vi "Periodic Tasks.vi"(8 "error in":errorcluster) -> ()   [LabVIEW 2016]
doc: "This VI runs in parallel to other tasks. It can contain as many user-defined periodic loops as you need. These can carry out PID or other sorts of timed response."
uses:
  Refname/Motors.ctl
  Refname/Sensors.ctl
  Refname/Queues.ctl
  <vilib>/Rock Robotics/WPI/DriverStation/WPI_DriverStationRobotMode2.ctl
  Refname/Refname to String (Motors).vi
  Robot Global Data.vi
  Refname/Refname to String (Sensors).vi
panel:
  in  "Low Sensitivity z":dbl=1.9 format="%#_13g"
  in  "Default Sensitivity z":dbl=1.6 format="%#_13g"
  in  "Low Sensitivity x & y":dbl=1.7 format="%#_13g"
  in  "Default Sensitivity x & y":dbl=1.4 format="%#_13g"
  out "error out":errorcluster
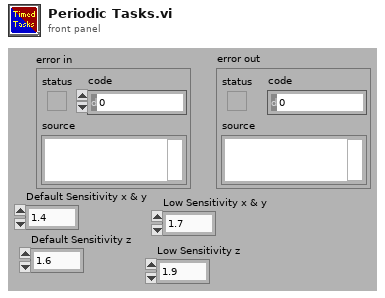
[diagram p1: front panel]
types:
  T1 = typedef "Queues.ctl" = enum16{"Log Queue"}
  T2 = typedef "Sensors.ctl" = enum16{"DIP 1", "DIP 2", "DIP 3", "DIP 4", "IMU", "HuskieBoard"}
  T3 = typedef "Motors.ctl" = enum16{"Wheel 1", "Swerve 1", "Wheel 2", "Swerve 2", "Wheel 3", "Swerve 3", "Wheel 4", "Swerve 4", "Climber"}
  T4 = typedef "WPI_MotorControlDeviceRef.ctl" = cluster{"DeviceStatus":errorcluster, "Type":T5, "PWM":cluster{"PWM Channel":T6, "DeadBand":T7}, "CAN":cluster{"Device Number":u8, "SetOutput VI Ref":variant, "GetOutput VI Ref":variant, "Enable VI Ref":variant, "Disable VI Ref":variant, "Data":variant}, "Invert":bool}
  T5 = typedef "WPI_MotorControlType.ctl" = enum16{"PWM", "CAN"}
  T6 = typedef "FPGA_DIOPWMChannel.ctl" = enum8{"PWM 0", "PWM 1", "PWM 2", "PWM 3", "PWM 4", "PWM 5", "PWM 6", "PWM 7", "PWM 8", "PWM 9", "PWM MXP 0", "PWM MXP 1", "PWM MXP 2", "PWM MXP 3", "PWM MXP 4", "PWM MXP 5", "PWM MXP 6", "PWM MXP 7", "PWM MXP 8", "PWM MXP 9", "Invalid"}
  T7 = typedef "WPI_PWMDeadband.ctl" = cluster{"Name":string, "maxPositivePwm":i32, "minPositivePwm":i32, "centerPwm":i32, "maxNegativePwm":i32, "minNegativePwm":i32, "angularRange":u16}
  T8 = typedef "WPI_SerialPortRef.ctl" = cluster{"DevStatus":errorcluster, "Serial Port Name":refnum<visa-resource-name>}
  T9 = enum8{"Don't Change", "Backlight On", "Backlight Off"}
  T10 = typedef "WPI_CANTalonSRX_GlobalStatus.ctl" = cluster{"Applied Throttle":dbl, "Module Enabled":bool, "CAN Error":errorcluster, "Closed Loop Error":dbl, "Forward Limit Switch Closed":bool, "Reverse Limit Switch Closed":bool, "Sensor Position":dbl, "Sensor Velocity":dbl, "Current":dbl, "Sticky Fault - Over Temp":bool, "Sticky Fault - Under Voltage":bool, "Sticky Fault - Forward Limit":bool, "Sticky Fault - Reverse Limit":bool, "Sticky Fault - Forward Soft Limit":bool, "Sticky Fault - Reverse Soft Limit":bool, "Brake is Enabled":bool, "Encoder Position":dbl, "Encoder Velocity":dbl, "Encoder Index Count":dbl, "Encoder A Pin State":bool, "Encoder B Pin State":bool, "Encoder Index Pin State":bool, "Analog In":dbl, "Analog In Velocity":dbl, "Temperature (C)":dbl, "Battery Voltage":dbl, "Control 5 Is Supported":bool, "Current Profile Slot Select":dbl, "Pos Div 8":bool, "Vel Div 4":bool, "Pulse Width Position":i32, "Pulse Width Velocity":i32, "Pulse Width Rise To Rise (us)":i32, "Pulse Width Rise To Fall (us)":i32, "Mot Prof Active Is Under Run":bool, "Mot Prof Active Has Under Run":bool, "Mot Prof Active Is Last":bool, "Mot Prof Active Velocity Only":bool, "Mot Prof Active Is Valid":bool, "Mot Prof Buffer Is Full":bool, "Mot Prof Active Profile Slot Select":i32, "Mot Prof NextID":i32, "Mot Prof Count":i32, "Mot Prof Active Velocity":dbl, "Mot Prof Active Position":dbl, "Mot Prof Output Enable":i32}
  T11 = cluster{"X":dbl, "Y":dbl, "Z":dbl, "B (Straight Drive)":bool, "T1 (Climber Up)":bool, "T2 (Climber Down)":bool, "Pinky Trigger (Low Sensitivity Drive)":bool, "Trigger Full Press (Reverse Drive)":bool, "LED Green":bool}
  T12 = typedef "WPI_DriverStationRobotMode2.ctl" = enum16{"Autonomous Disabled", "Autonomous Enabled", "Teleop Disabled", "Teleop Enabled", "Disconnected", "Finish", "Test Disabled", "Test Enabled", "Emergency Stopped"}
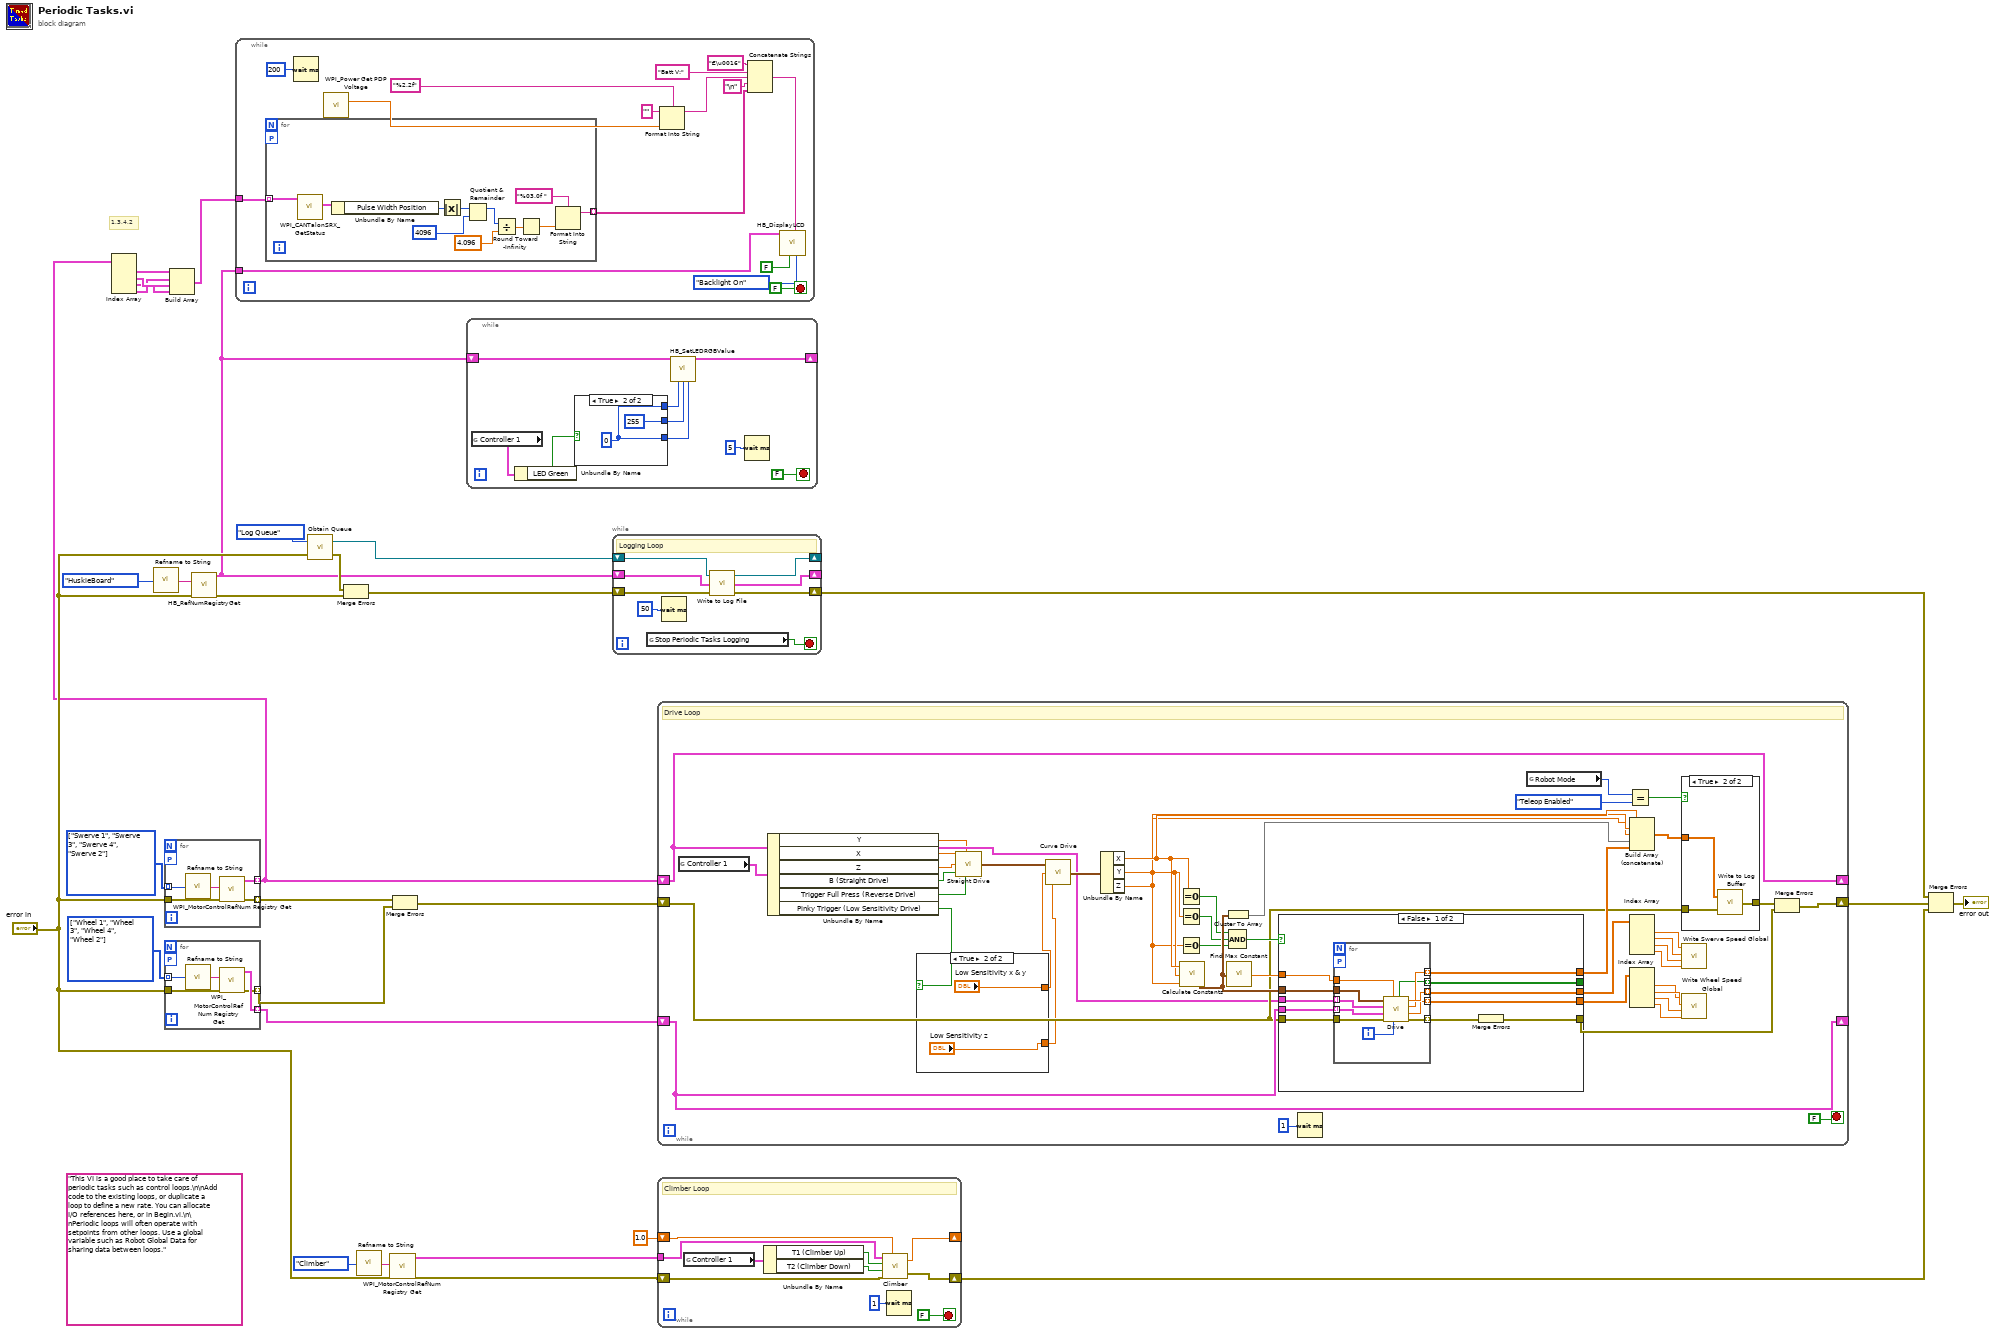
[diagram p0: block diagram]
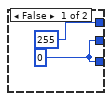
[diagram p2: hidden frame]
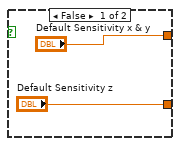
[diagram p3: hidden frame]
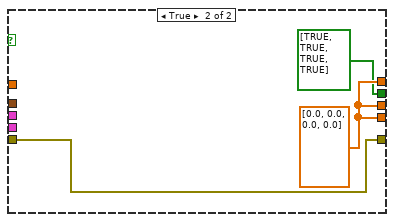
[diagram p4: hidden frame]
diagram:
  w28 = T3[] [enum."Wheel 1", enum."Wheel 3", enum."Wheel 4", enum."Wheel 2"] items=["Wheel 1", "Swerve 1", "Wheel 2", "Swerve 2", "Wheel 3", "Swerve 3", "Wheel 4", "Swerve 4", "Climber"]
  w29 = T3[] [enum."Swerve 1", enum."Swerve 3", enum."Swerve 4", enum."Swerve 2"] items=["Wheel 1", "Swerve 1", "Wheel 2", "Swerve 2", "Wheel 3", "Swerve 3", "Wheel 4", "Swerve 4", "Climber"]
  (unwired) "This VI is a good place to take care of periodic tasks such as control loops.\n\nAdd code to the existing loops, or duplicate a loop to define a new rate. You can allocate I/O references here, or in Begin.vi.\n\nPeriodic loops will often operate with setpoints from other loops. Use a global variable such as Robot Global Data for sharing data between loops."
  # "1,3,4,2"
  n1 = call-poly "Refname to String.vi"("Enum"=Sensors."HuskieBoard") -> ("String"=w17:string)
  n2 = for {
    tunnel: [w35] -> w6 mode=indexing
    tunnel: w29 -> [w33] mode=indexing
    workers-P: _ -> [_]
    tunnel: "error in" -> [w32]
    tunnel: [w31] -> w26 mode=indexing
    n3 = call-poly "Refname to String.vi"("Enum"=w33) -> ("String"=w34:string)
    n4 = call <vilib>:"WPI_MotorControlRefNum Registry Get.vi"("error in (no error)"=w32, "refnum name"=w34) -> ("error out"=w31:errorcluster, "MotorControlDevRef"=w35:T4)  [unwired: 8 in]
  }
  n5 = Index Array(array=w6) -> (element #1=w5:T4, element #2=w4:T4, element #3=w3:T4, element #4=w2:T4)  [unwired: 4 in]
  n6 = for {
    tunnel: [w40] -> w30 mode=indexing
    tunnel: w28 -> [w38] mode=indexing
    workers-P: _ -> [_]
    tunnel: "error in" -> [w37]
    tunnel: [w36] -> w25 mode=indexing
    n7 = call-poly "Refname to String.vi"("Enum"=w38) -> ("String"=w39:string)
    n8 = call <vilib>:"WPI_MotorControlRefNum Registry Get.vi"("error in (no error)"=w37, "refnum name"=w39) -> ("error out"=w36:errorcluster, "MotorControlDevRef"=w40:T4)  [unwired: 8 in]
  }
  n9 = Build Array(w5, w2, w4, w3) -> (w1:T4[])
  n10 = call <vilib>:"HB_RefNumRegistryGet.vi"("refnum name"=w17, "error in (no error)"="error in") -> ("HBDevRef"=w7:T8, "error out"=w11:errorcluster)  [unwired: 12 in]
  n11 = while {
    tunnel: w7 -> [w53]
    tunnel: w1 -> [w42]
    stop <- FALSE stop-if-true
    n12 = for {
      tunnel: w42 -> [w66] mode=indexing
      workers-P: _ -> [_]
      tunnel: [w57] -> w41 mode=indexing
      n13 = call <vilib>:"WPI_CANTalonSRX_GetStatus.vi"("CAN Talon SRX Ref"=w66) -> ("Talon SRX Status"=w65:T10)  [unwired: 8 in, 2 out]
      n14 = Unbundle By Name(w65) -> ("Pulse Width Position"=w64:i32)
      n15 = Absolute Value(x=w64) -> (abs(x)=w63:i32)
      n16 = Quotient & Remainder(x=w63, y=4096) -> (x-y*floor(x/y)=w56:i32)  [unwired: 1 out]
      n17 = Divide(x=w56, y=4.096) -> (x/y=w60:dbl)
      n18 = Round Toward -Infinity(1:w60) -> (0:w58:dbl)
      n19 = Format Into String(format string="%03.0f ", w58) -> (resulting string=w57:string)  [unwired: 2 in, 1 out]
    }
    n20 = Wait (ms)(milliseconds to wait=u32 200) -> ()  [unwired: 1 out]
    n21 = call <vilib>:"WPI_Power Get PDP Voltage.vi"() -> ("voltage (V)"=w49:dbl)  [unwired: 14 in, 1 out]
    n22 = Format Into String(format string="%2.2f", initial string="", w49) -> (resulting string=w47:string)  [unwired: 1 in, 1 out]
    n23 = Concatenate Strings("€\u0016" ("string"), "Batt V:" ("string"), w47, "\n" ("string"), w41) -> (w52:string)
    n24 = call <vilib>:"HB_DisplayLCD.vi"("LCD Backlight"=T9."Backlight On", "Clear LCD Display"=FALSE, "Display String"=w52, "HBDeviceRef"=w53) -> ()  [unwired: 6 in, 2 out]
  }
  n25 = call "Obtain Queue.vi"("error in"="error in", "Queue"=Queues."Log Queue") -> ("error out"=w12:errorcluster, "Queue Ref"=w14:refnum<queue>)
  n26 = Merge Errors(w12, w11) -> (w13:errorcluster)
  n27 = call-poly "Refname to String.vi"("Enum"=Motors."Climber") -> ("String"=w24:string)
  n28 = call <vilib>:"WPI_MotorControlRefNum Registry Get.vi"("error in (no error)"="error in", "refnum name"=w24) -> ("error out"=w21:errorcluster, "MotorControlDevRef"=w22:T4)  [unwired: 8 in]
  n29 = Merge Errors(w26, w25) -> (w19:errorcluster)
  n30 = while {
    shift-right: [w74] -> _
    shift-left: w7 -> [w75]
    stop <- FALSE stop-if-true
    n31 = global read "Robot Global Data.vi" "Controller 1"() -> (w69:T11)
    n32 = Unbundle By Name(w69) -> ("LED Green"=w68:bool)
    n33 = case shown="True" w68 {
      tunnel: [255 w78] -> w73
      tunnel: [w76 255] -> w72
      tunnel: [w76 w78] -> w71
      frame False {
        w76 = 0
      }
      frame True {
        w78 = 0
      }
    }
    n34 = call <vilib>:"HB_SetLEDRGBValue.vi"("HBDevRef"=w75, "Red"=w73, "Green"=w72, "Blue"=w71) -> ("HBDevRef"=w74:T8)  [unwired: 10 in, 1 out]
    n35 = Wait (ms)(milliseconds to wait=u32 5) -> ()  [unwired: 1 out]
  }
  n36 = while {
    shift-right: [w85] -> _
    shift-left: w14 -> [w86]
    shift-right: [w83] -> _
    shift-left: w7 -> [w84]
    shift-right: [w81] -> w10
    shift-left: w13 -> [w82]
    stop <- w87 stop-if-true
    # "Logging Loop"
    n37 = global read "Robot Global Data.vi" "Stop Periodic Tasks Logging"() -> (w87:bool)
    n38 = Wait (ms)(milliseconds to wait=u32 50) -> ()  [unwired: 1 out]
    n39 = call "Write to Log File.vi"("error in"=w82, "HBDevRef"=w84, "Log Queue"=w86) -> ("error out"=w81:errorcluster, "HBDevRef"=w83:T8, "Log Queue"=w85:refnum<queue>)
  }
  n40 = while {
    shift-right: [w97] -> _
    shift-left: w6 -> [w97]
    shift-right: [w129] -> _
    shift-left: w30 -> [w129]
    shift-right: [w112] -> w9
    shift-left: w19 -> [w98]
    stop <- FALSE stop-if-true
    # "Drive Loop"
    n41 = global read "Robot Global Data.vi" "Controller 1"() -> (w93:T11)
    n42 = Unbundle By Name(w93) -> ("Y"=w89:dbl, "X"=w88:dbl, "Z"=w90:dbl, "B (Straight Drive)"=w91:bool, "Trigger Full Press (Reverse Drive)"=w92:bool, "Pinky Trigger (Low Sensitivity Drive)"=w96:bool)
    n43 = case shown="True" w96 {
      tunnel: ["Default Sensitivity x & y" "Low Sensitivity x & y"] -> w95
      tunnel: ["Default Sensitivity z" "Low Sensitivity z"] -> w94
      frame False {
      }
      frame True {
      }
    }
    n44 = call "Straight Drive.vi"("X"=w88, "Y"=w89, "Z"=w90, "Straight?"=w91, "Reverse?"=w92) -> ("Axes Magnitudes"=w99:cluster{"X":dbl, "Y":dbl, "Z":dbl})
    n45 = call "Curve Drive.vi"("z exponent"=w94, "x & y exponent"=w95, "Axes Magnitudes"=w99) -> ("Axes Magnitudes"=w100:cluster{"X":dbl, "Y":dbl, "Z":dbl})
    n46 = Unbundle By Name(w100) -> ("X"=w103:dbl, "Y"=w102:dbl, "Z"=w101:dbl)
    n47 = Equal To 0?(x=w103) -> (x = 0?=w120:bool)
    n48 = Equal To 0?(x=w102) -> (x = 0?=w119:bool)
    n49 = Equal To 0?(x=w101) -> (x = 0?=w118:bool)
    n50 = call "Calculate Constants.vi"("Z"=w101, "Y"=w102, "X"=w103) -> ("constants cluster"=w122:cluster{"a":dbl, "b":dbl, "c":dbl, "d":dbl})
    n51 = Cluster To Array(cluster=w122) -> (array=w108:dbl[])
    n52 = call "Find Max Constant.vi"("constants"=w122) -> ("Max or 1"=w121:dbl)
    n53 = Compound Arithmetic op=AND(w120, w119, w118) -> (w117:bool)
    n54 = case shown="False" w117 {
      tunnel: w129 -> [w146 _]
      tunnel: [w145 w160] -> w126
      tunnel: [w144 w160] -> w125
      tunnel: w98 -> [w143 w159]
      tunnel: w97 -> [w142 _]
      tunnel: w122 -> [w141 _]
      tunnel: w121 -> [w140 _]
      tunnel: [w139 w160] -> w109
      tunnel: [w138 w159] -> w104
      tunnel: [w136 bool[] [TRUE, TRUE, TRUE, TRUE]] -> _
      frame False {
        n55 = for {
          tunnel: w142 -> [w148] mode=indexing
          tunnel: w146 -> [w157] mode=indexing
          tunnel: [w156] -> w145 mode=indexing
          tunnel: [w155] -> w144 mode=indexing
          tunnel: w143 -> [w154]
          tunnel: [w150] -> w137 mode=indexing
          tunnel: w141 -> [w153]
          tunnel: w140 -> [w152]
          tunnel: [w149] -> w139 mode=indexing
          workers-P: _ -> [_]
          tunnel: [w147] -> w136 mode=indexing
          i -> [w151]
          n56 = call "Drive.vi"("Index"=w151, "Max Speed or 1"=w152, "error in"=w154, "Wheel DevRef"=w157, "Swerve DevRef"=w148, "constants"=w153) -> ("error out"=w150:errorcluster, "Wheel Speed"=w155:dbl, "Setpoint"=w149:dbl, "Swerve Speed"=w156:dbl, "Reverse?"=w147:bool)  [unwired: 1 in]
        }
        n57 = Merge Errors(w137) -> (w138:errorcluster)
      }
      frame True {
        w160 = dbl[] [0.0, 0.0, 0.0, 0.0]
      }
    }
    n58 = Wait (ms)(milliseconds to wait=u32 1) -> ()  [unwired: 1 out]
    n59 = global read "Robot Global Data.vi" "Robot Mode"() -> (w105:T12)
    n60 = Equal?(x=w105, y=WPI_DriverStationRobotMode2."Teleop Enabled" ("Robot Mode")) -> (x = y?=w107:bool)
    n61 = Build Array (concatenate)(w103, w102, w101, w108, w109) -> (w110:dbl[])
    n62 = Index Array(array=w126) -> (element #1=w116:dbl, element #2=w115:dbl, element #3=w114:dbl, element #4=w113:dbl)  [unwired: 4 in]
    n63 = Index Array(array=w125) -> (element #1=w127:dbl, element #2=w128:dbl, element #3=w124:dbl, element #4=w123:dbl)  [unwired: 4 in]
    n64 = case shown="True" w107 {
      tunnel: w110 -> [_ w162]
      tunnel: [w161 w164] -> w111
      tunnel: w98 -> [w161 w163]
      frame False {
      }
      frame True {
        n65 = call "Write to Log Buffer.vi"("error in"=w163, "array of values"=w162) -> ("error out"=w164:errorcluster)
      }
    }
    n66 = call "Write Swerve Speed Global.vi"("Swerve 4"=w113, "Swerve 3"=w114, "Swerve 2"=w115, "Swerve 1"=w116) -> ()
    n67 = call "Write Wheel Speed Global.vi"("Wheel 4"=w123, "Wheel 3"=w124, "Wheel 2"=w128, "Wheel 1"=w127) -> ()
    n68 = Merge Errors(w111, w104) -> (w112:errorcluster)
  }
  n69 = while {
    tunnel: w22 -> [w170]
    shift-right: [w169] -> _
    shift-left: 1.0 ("Multiplier") -> [w168]
    shift-right: [w165] -> w8
    shift-left: w21 -> [w171]
    stop <- FALSE stop-if-true
    # "Climber Loop"
    n70 = global read "Robot Global Data.vi" "Controller 1"() -> (w174:T11)
    n71 = Unbundle By Name(w174) -> ("T1 (Climber Up)"=w173:bool, "T2 (Climber Down)"=w172:bool)
    n72 = call "Climber.vi"("Climber Dev Ref"=w170, "Forward Climb"=w173, "Backwards Climb"=w172, "error in"=w171, "Current Multiplier"=w168) -> ("Multiplier"=w169:dbl, "error out"=w165:errorcluster)
    n73 = Wait (ms)(milliseconds to wait=u32 1) -> ()  [unwired: 1 out]
  }
  n74 = Merge Errors(w10, w9, w8) -> (→"error out":errorcluster)
